vi "wrl_import_Ex.vi"() -> ()   [LabVIEW 2020]
uses:
  <vilib>/picture/3D Picture Control/Object/Create Object (name).vi
  <vilib>/Utility/file.llb/Read Delimited Spreadsheet (string).vi
  <vilib>/picture/3D Picture Control/NI_3D Picture Control.lvlib
panel:
  out "Waveform Chart":cluster{"x_axis":dbl, "z_axis":dbl}(graph)
  out "XY Graph":cluster{dbl[], dbl[]}(graph)
  out "deleted portion":string[](array[string])
  out "3D 그림":refnum<vi>(3d-picture)
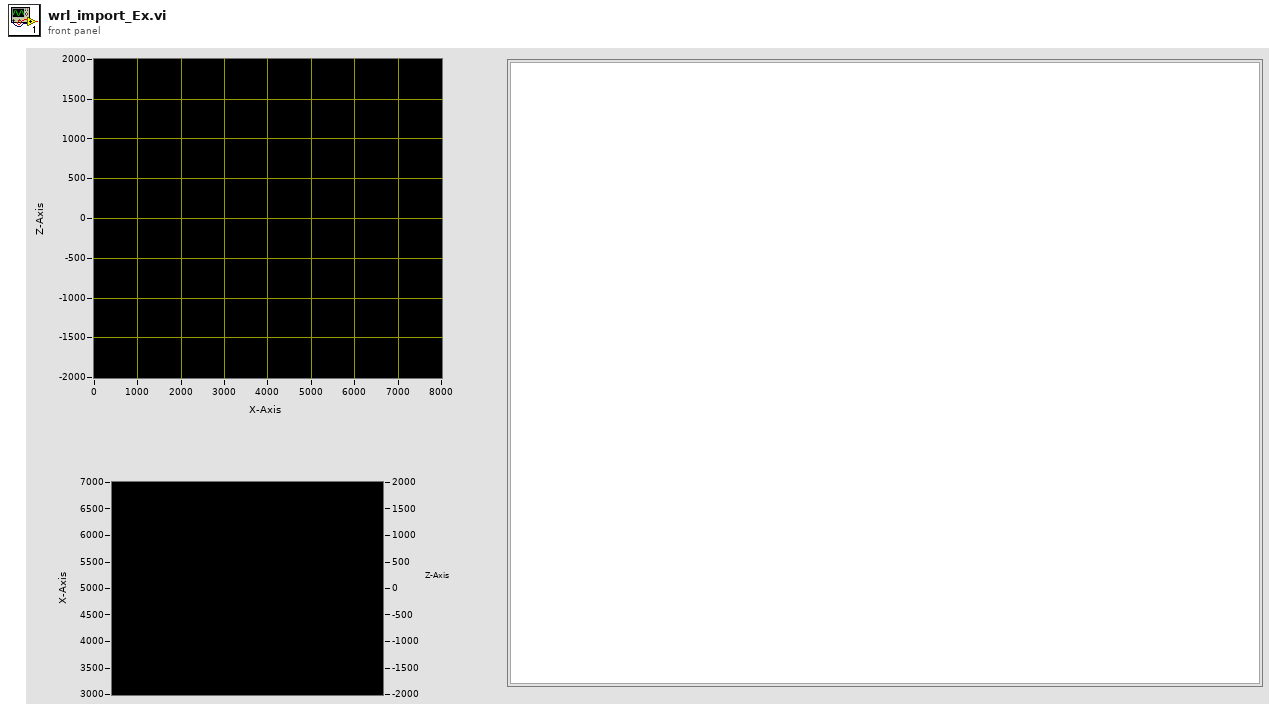
[diagram p1: front panel]
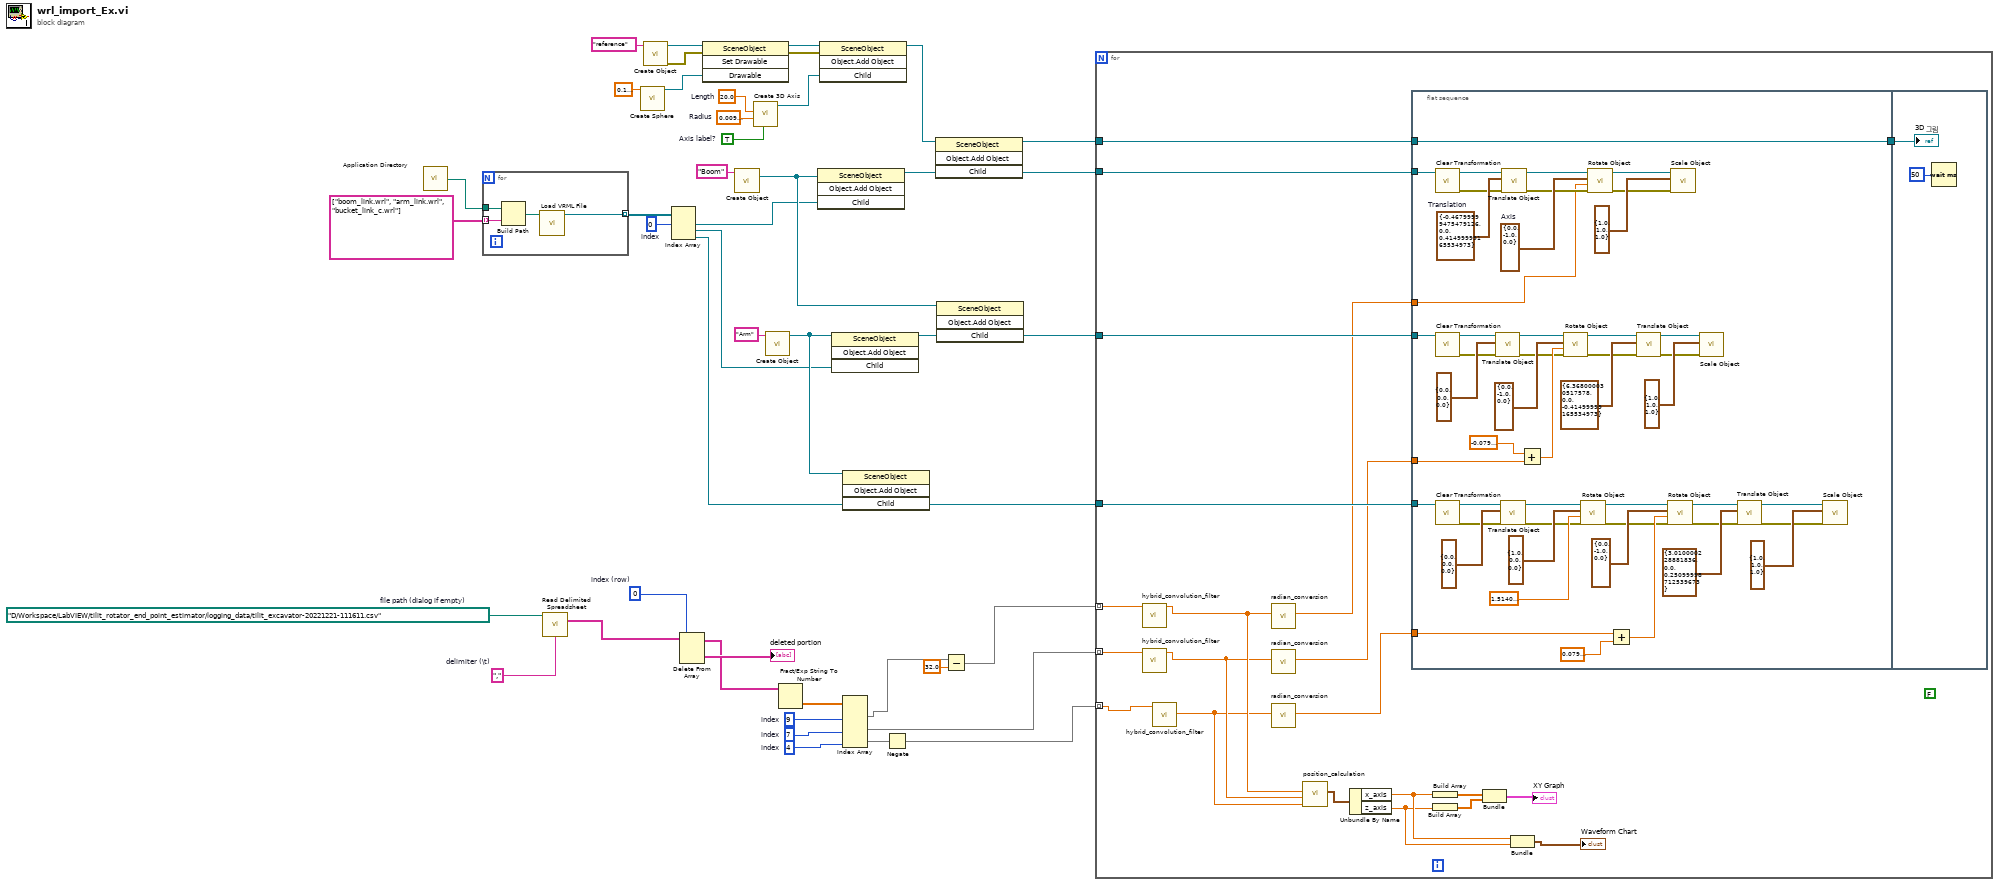
[diagram p0: block diagram]
diagram:
  w7 = 4  # index
  w8 = 7  # index
  w9 = 9  # index
  w12 = ","  # delimiter (\t)
  w14 = 0  # index (row)
  w16 = path "D:/Workspace/LabVIEW/tilit_rotator_end_point_estimator/logging_data/tilit_excavator-20221221-111611.csv"  # file path (dialog if empty)
  w23 = 0  # index
  w31 = TRUE  # Axis label?
  w32 = sgl 0.01  # Radius
  w33 = sgl 20.0  # Length
  n1 = call <vilib>:"Application Directory.vi"() -> ("Application Directory"=w24:path)
  n2 = for {
    tunnel: string[] ["boom_link.wrl", "arm_link.wrl", "bucket_link_c.wrl"] -> [w49] mode=indexing
    tunnel: w24 -> [w48]
    tunnel: [w46] -> w21 mode=indexing
    n3 = Build Path(base path=w48, name or relative path=w49) -> (appended path=w47:path)
    n4 = call <vilib>:"Load VRML File.vi"("Path"=w47) -> ("Scene:Read Scene File"=w46:refnum<vi>)  [unwired: 9 in, 1 out]
  }
  n5 = call-poly <vilib>:"Read Delimited Spreadsheet.vi"("file path (dialog if empty)"=w16, "delimiter (\\t)"=w12) -> ("all rows"=w15:string[][])  [unwired: 8 in, 5 out]
  n6 = call <vilib>:"Create Sphere.vi"("Radius"=sgl 0.1) -> ("New Sphere Refnum"=w42:refnum<vi>)  [unwired: 9 in, 1 out]
  n7 = call-poly <vilib>:"Create Object.vi"("Name"="reference") -> ("error out"=w18:errorcluster, "Scene:New Object"=w43:refnum<vi>)  [unwired: 9 in]
  n8 = Index Array "Index Array"(array=w21, index #1=w23) -> (element #1=w22:refnum<vi>, element #2=w20:refnum<vi>, element #3=w19:refnum<vi>)  [unwired: 2 in]
  n9 = Delete From Array(array=w15, index (row)=w14) -> (deleted portion=→"deleted portion":string[], array with subset deleted=w11:string[][])  [unwired: 2 in]
  n10 = invoke class="SceneObject" method="Set Drawable"(reference=w43, error in=w18, "Drawable"=w42) -> (reference out=w35:refnum<vi>, error out=w17:errorcluster)  [unwired: 1 in, 2 out]
  n11 = call-poly <vilib>:"Create Object.vi"("Name"="Boom") -> ("Scene:New Object"=w38:refnum<vi>)  [unwired: 9 in, 1 out]
  n12 = call <vilib>:"Create 3D Axis.vi"("Axis label?"=w31, "Radius"=w32, "Length"=w33) -> ("New Object Refnum"=w34:refnum<vi>)  [unwired: 7 in, 1 out]
  n13 = call-poly <vilib>:"Create Object.vi"("Name"="Arm") -> ("Scene:New Object"=w28:refnum<vi>)  [unwired: 9 in, 1 out]
  n14 = Fract/Exp String To Number(string=w11) -> (number=w10:dbl[][])  [unwired: 3 in, 1 out]
  n15 = invoke class="SceneObject" method="Object.Add Object"(reference=w38, "Child"=w22) -> (reference out=w40:refnum<vi>)  [unwired: 2 in, 3 out]
  n16 = invoke class="SceneObject" method="Object.Add Object"(reference=w35, error in=w17, "Child"=w34) -> (reference out=w36:refnum<vi>)  [unwired: 1 in, 3 out]
  n17 = invoke class="SceneObject" method="Object.Add Object"(reference=w28, "Child"=w20) -> (reference out=w29:refnum<vi>)  [unwired: 2 in, 3 out]
  n18 = invoke class="SceneObject" method="Object.Add Object"(reference=w28, "Child"=w19) -> ("Child"=w26:refnum<vi>)  [unwired: 2 in, 3 out]
  n19 = Index Array(array=w10, index (col) #1=w9, index (col) #2=w8, index (col) #3=w7) -> (element #1=w2:dbl[], element #2=w6:dbl[], element #3=w5:dbl[])  [unwired: 3 in]
  n20 = Negate(x=w5) -> (-x=w4:dbl[])
  n21 = invoke class="SceneObject" method="Object.Add Object"(reference=w36, "Child"=w40) -> (reference out=w41:refnum<vi>, "Child"=w37:refnum<vi>)  [unwired: 2 in, 2 out]
  n22 = invoke class="SceneObject" method="Object.Add Object"(reference=w38, "Child"=w29) -> ("Child"=w27:refnum<vi>)  [unwired: 2 in, 3 out]
  n23 = Subtract(x=w2, y=32.0) -> (x-y=w1:dbl[])
  n24 = for {
    tunnel: w41 -> [w70]
    tunnel: w37 -> [w68]
    tunnel: w27 -> [w67]
    tunnel: w26 -> [w66]
    tunnel: w1 -> [w55] mode=indexing
    tunnel: w6 -> [w54] mode=indexing
    tunnel: w4 -> [w53] mode=indexing
    (unwired) FALSE
    n25 = call "hybrid_convolution_filter.vi"("input"=w55) -> ("output"=w62:dbl)  [unwired: 10 in]
    n26 = call "hybrid_convolution_filter.vi"("input"=w54) -> ("output"=w61:dbl)  [unwired: 10 in]
    n27 = call "hybrid_convolution_filter.vi"("input"=w53) -> ("output"=w60:dbl)  [unwired: 10 in]
    n28 = call "radian_conversion.vi"("input"=w62) -> ("output"=w65:dbl)  [unwired: 10 in]
    n29 = call "radian_conversion.vi"("input"=w61) -> ("output"=w64:dbl)  [unwired: 10 in]
    n30 = call "radian_conversion.vi"("input"=w60) -> ("output"=w63:dbl)  [unwired: 10 in]
    n31 = call "position_calculation.vi"("bucket_angle"=w60, "arm_angle"=w61, "boom_angle"=w62) -> ("end_point"=w59:cluster{"x_axis":dbl, "z_axis":dbl})  [unwired: 8 in]
    n32 = Unbundle By Name(w59) -> ("x_axis"=w52:dbl, "z_axis"=w51:dbl)
    n33 = flat-sequence {
      tunnel: w70 -> [w118]
      tunnel: [w118] -> w69
      tunnel: w68 -> [w116]
      tunnel: w67 -> [w102]
      tunnel: w66 -> [w95]
      tunnel: w65 -> [w73]
      tunnel: w64 -> [w72]
      tunnel: w63 -> [w71]
      tunnel: w69 -> [w119]
      frame #0 {
        w117 = cluster{"X":sgl, "Y":sgl, "Z":sgl} {"X"=-0.468, "Y"=0.0, "Z"=0.415}  # Translation
        w112 = cluster{"X":sgl, "Y":sgl, "Z":sgl} {"X"=0.0, "Y"=-1.0, "Z"=0.0}  # Axis
        n34 = call <vilib>:"Clear Transformation.vi"("Object Refnum In"=w116) -> ("error out"=w85:errorcluster, "Object Refnum Out"=w115:refnum<vi>)  [unwired: 9 in]
        n35 = call <vilib>:"Clear Transformation.vi"("Object Refnum In"=w102) -> ("error out"=w77:errorcluster, "Object Refnum Out"=w110:refnum<vi>)  [unwired: 9 in]
        n36 = call <vilib>:"Clear Transformation.vi"("Object Refnum In"=w95) -> ("error out"=w83:errorcluster, "Object Refnum Out"=w101:refnum<vi>)  [unwired: 9 in]
        n37 = call <vilib>:"Translate Object.vi"("error in (no error)"=w77, "Translation"=cluster{"X":sgl, "Y":sgl, "Z":sgl} {"X"=0.0, "Y"=0.0, "Z"=0.0}, "Scene.Object In"=w110) -> ("error out"=w76:errorcluster, "Scene.Object Out"=w108:refnum<vi>)  [unwired: 7 in]
        n38 = call <vilib>:"Translate Object.vi"("error in (no error)"=w83, "Translation"=cluster{"X":sgl, "Y":sgl, "Z":sgl} {"X"=0.0, "Y"=0.0, "Z"=0.0}, "Scene.Object In"=w101) -> ("error out"=w82:errorcluster, "Scene.Object Out"=w89:refnum<vi>)  [unwired: 7 in]
        n39 = call <vilib>:"Translate Object.vi"("error in (no error)"=w85, "Translation"=w117, "Scene.Object In"=w115) -> ("error out"=w84:errorcluster, "Scene.Object Out"=w113:refnum<vi>)  [unwired: 7 in]
        n40 = Add(x=-0.07999999821186066 ("y"), y=w72) -> (x+y=w93:dbl)
        n41 = call <vilib>:"Rotate Object.vi"("error in (no error)"=w76, "Angle"=w93, "Axis"=cluster{"X":sgl, "Y":sgl, "Z":sgl} {"X"=0.0, "Y"=-1.0, "Z"=0.0}, "Scene.Object In"=w108) -> ("error out"=w75:errorcluster, "Scene.Object Out"=w104:refnum<vi>)  [unwired: 6 in]
        n42 = call <vilib>:"Rotate Object.vi"("error in (no error)"=w82, "Angle"=sgl 1.514, "Axis"=cluster{"X":sgl, "Y":sgl, "Z":sgl} {"X"=1.0, "Y"=0.0, "Z"=0.0}, "Scene.Object In"=w89) -> ("error out"=w81:errorcluster, "Scene.Object Out"=w87:refnum<vi>)  [unwired: 6 in]
        n43 = call <vilib>:"Rotate Object.vi"("error in (no error)"=w84, "Angle"=w73, "Axis"=w112, "Scene.Object In"=w113) -> ("error out"=w78:errorcluster, "Scene.Object Out"=w111:refnum<vi>)  [unwired: 6 in]
        n44 = Add(x=w71, y=0.07999999821186066) -> (x+y=w91:dbl)
        n45 = call <vilib>:"Translate Object.vi"("error in (no error)"=w75, "Translation"=cluster{"X":sgl, "Y":sgl, "Z":sgl} {"X"=6.368, "Y"=0.0, "Z"=-0.415}, "Scene.Object In"=w104) -> ("error out"=w74:errorcluster, "Scene.Object Out"=w103:refnum<vi>)  [unwired: 7 in]
        n46 = call <vilib>:"Rotate Object.vi"("error in (no error)"=w81, "Angle"=w91, "Axis"=cluster{"X":sgl, "Y":sgl, "Z":sgl} {"X"=0.0, "Y"=-1.0, "Z"=0.0}, "Scene.Object In"=w87) -> ("error out"=w80:errorcluster, "Scene.Object Out"=w97:refnum<vi>)  [unwired: 6 in]
        n47 = call <vilib>:"Scale Object.vi"("error in (no error)"=w78, "Scale"=cluster{"X":sgl, "Y":sgl, "Z":sgl} {"X"=1.0, "Y"=1.0, "Z"=1.0}, "Scene.Object In"=w111) -> ()  [unwired: 7 in, 2 out]
        n48 = call <vilib>:"Scale Object.vi"("error in (no error)"=w74, "Scale"=cluster{"X":sgl, "Y":sgl, "Z":sgl} {"X"=1.0, "Y"=1.0, "Z"=1.0}, "Scene.Object In"=w103) -> ()  [unwired: 7 in, 2 out]
        n49 = call <vilib>:"Translate Object.vi"("error in (no error)"=w80, "Translation"=cluster{"X":sgl, "Y":sgl, "Z":sgl} {"X"=3.0100002, "Y"=0.0, "Z"=0.251}, "Scene.Object In"=w97) -> ("error out"=w79:errorcluster, "Scene.Object Out"=w96:refnum<vi>)  [unwired: 7 in]
        n50 = call <vilib>:"Scale Object.vi"("error in (no error)"=w79, "Scale"=cluster{"X":sgl, "Y":sgl, "Z":sgl} {"X"=1.0, "Y"=1.0, "Z"=1.0}, "Scene.Object In"=w96) -> ()  [unwired: 7 in, 2 out]
      }
      frame #1 {
        n51 = Wait (ms)(milliseconds to wait=u32 50 ("대기 시간 (ms)")) -> ()  [unwired: 1 out]
        "3D 그림" <- w119
      }
    }
    n52 = Build Array(w52) -> (w58:dbl[])
    n53 = Build Array(w51) -> (w57:dbl[])
    n54 = Bundle(w58, w57) -> (→"XY Graph":cluster{dbl[], dbl[]})  [unwired: 1 in]
    n55 = Bundle("x_axis"=w52, "z_axis"=w51) -> (→"Waveform Chart":cluster{"x_axis":dbl, "z_axis":dbl})  [unwired: 1 in]
  }
